vi "FCE_TS_Action_ReadExcelSettings.vi"(8 "error in":errorcluster, 9 "WriteEnums":bool, 10 "ExcelVisible":bool=TRUE, 11 "ExcelFile":path=path "B:/Kirschenhofer/FutureE/FCE_TS/doc/Ansteuerung_Sensoren_Aktoren.xlsx") -> (0 "error out":errorcluster)   [LabVIEW 2017]
panel:
  in  "TDefPath":path=path "B:/Kirschenhofer/FutureE/FCET/Software/01_SourceCode/FCET_ProjectLibs"
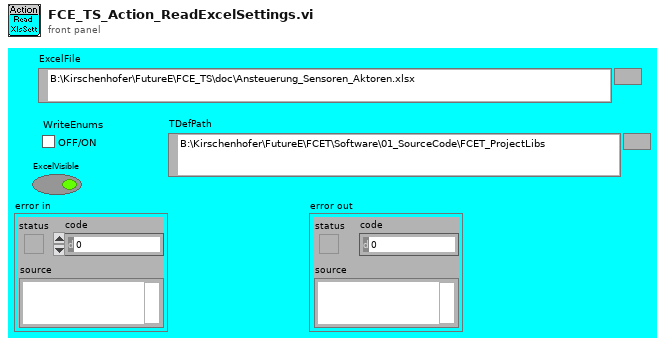
[diagram p1: front panel]
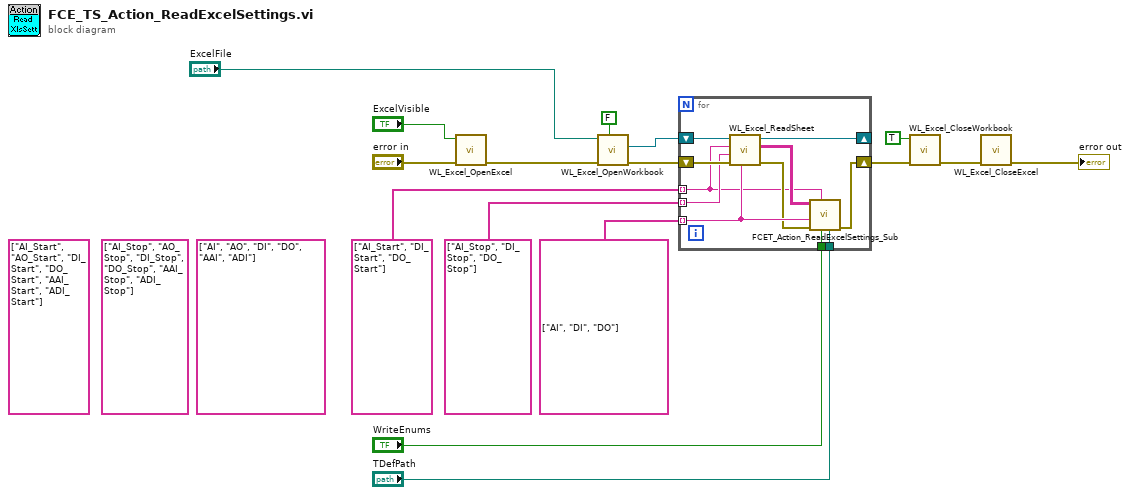
[diagram p0: block diagram]
diagram:
  (unwired) string[] ["AI_Stop", "AO_Stop", "DI_Stop", "DO_Stop", "AAI_Stop", "ADI_Stop"]
  (unwired) string[] ["AI_Start", "AO_Start", "DI_Start", "DO_Start", "AAI_Start", "ADI_Start"]
  (unwired) string[] ["AI", "AO", "DI", "DO", "AAI", "ADI"]
  n1 = call "WL_Excel_OpenExcel.vi"("error in"="error in", "Visible"="ExcelVisible") -> ("error out"=w15:errorcluster)  [unwired: 7 in, 2 out]
  n2 = call "WL_Excel_OpenWorkbook.vi"("ProgressBar"=FALSE, "error in"=w15, "Excel File Path"="ExcelFile") -> ("error out"=w14:errorcluster, "Workbook"=w6:refnum<k7>)  [unwired: 6 in, 1 out]
  n3 = for {
    shift-right: [w20] -> w13
    shift-left: w14 -> [w27]
    shift-right: [w25] -> _
    shift-left: w6 -> [w26]
    tunnel: string[] ["AI", "DI", "DO"] -> [w22] mode=indexing
    tunnel: string[] ["AI_Start", "DI_Start", "DO_Start"] -> [w17] mode=indexing
    tunnel: string[] ["AI_Stop", "DI_Stop", "DO_Stop"] -> [w24] mode=indexing
    tunnel: "WriteEnums" -> [w19]
    tunnel: "TDefPath" -> [w18]
    n4 = call "WL_Excel_ReadSheet.vi"("SheetName"=w22, "error in"=w27, "CellStop"=w24, "CellStart"=w17, "Workbook"=w26) -> ("error out"=w21:errorcluster, "CellValues"=w23:string[][], "Workbook Out"=w25:refnum<k7>)  [unwired: 4 in]
    n5 = call "FCET_Action_ReadExcelSettings_Sub.vi"("TDefPath"=w18, "WriteEnums"=w19, "Start_Cell"=w17, "error in"=w21, "Sheet"=w22, "Data"=w23) -> ("error out"=w20:errorcluster)  [unwired: 5 in]
  }
  n6 = call "WL_Excel_CloseWorkbook.vi"("error in"=w13, "SaveChanges"=TRUE) -> ("error out"=w9:errorcluster)  [unwired: 9 in]
  n7 = call "WL_Excel_CloseExcel.vi"("error in"=w9) -> ("error out"=→"error out":errorcluster)  [unwired: 10 in]
